vi "Secondary Moniter.vi"() -> ()   [LabVIEW 2018]
uses:
  <vilib>/Rock Robotics/Network Tables/NT Read Number.vi
  <vilib>/Rock Robotics/Network Tables/NT Read Boolean.vi
  <vilib>/Rock Robotics/Network Tables/NT Read Boolean Array.vi
panel:
  out "Boolean 10":bool
  out "Boolean 9":bool
  out "Boolean 8":bool
  out "Boolean 7":bool
  out "Boolean 6":bool
  out "Boolean 5":bool
  out "Boolean 4":bool
  out "Boolean 3":bool
  out "Boolean 2":bool
  out "Boolean":bool
  out "XY Graph":cluster{"Y":dbl[], "Y":dbl[]}[](graph)
  out "Low Gear":bool
  out "High Gear":bool
  out "Climber":bool
  out "Robot Centric":bool
  out "Field Centric":bool
  out "Tracks":bool caption="Brakes"
  out "Match Time":string
  out "Camera Image 2":T1(plugin-control)
  out "PSI":dbl(slide) scale=0.0..160.0
  out "Gyro":cluster{dbl, dbl}(knob) scale=0.0..360.0 scale format="%#.3g"
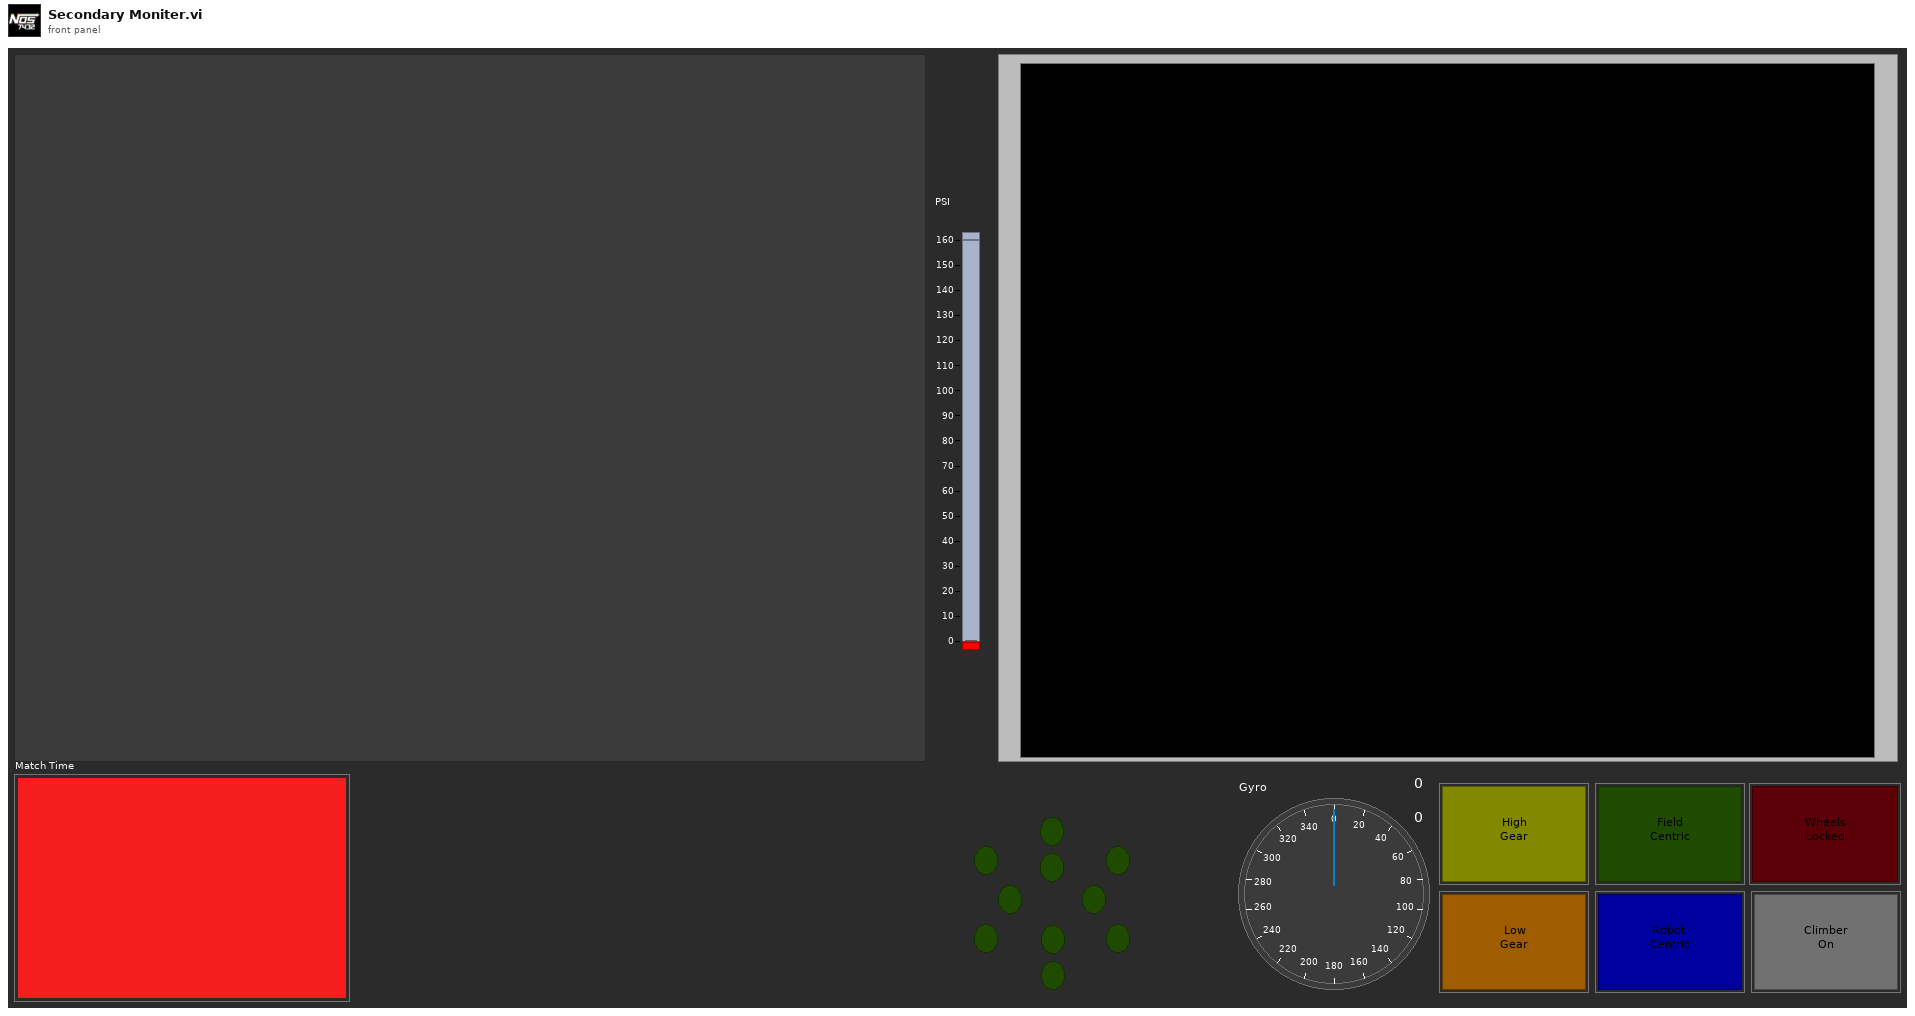
[diagram p1: front panel]
types:
  T1 = typedef "IMAQ Image.ctl" = refnum<image>
  T2 = typedef "LVDateTimeRec.ctl" = cluster{"fractional second":dbl, "second":i32, "minute":i32, "hour":i32, "day of month":i32, "month":i32, "year":i32, "day of week":i32, "day of year":i32, "DST":i32}
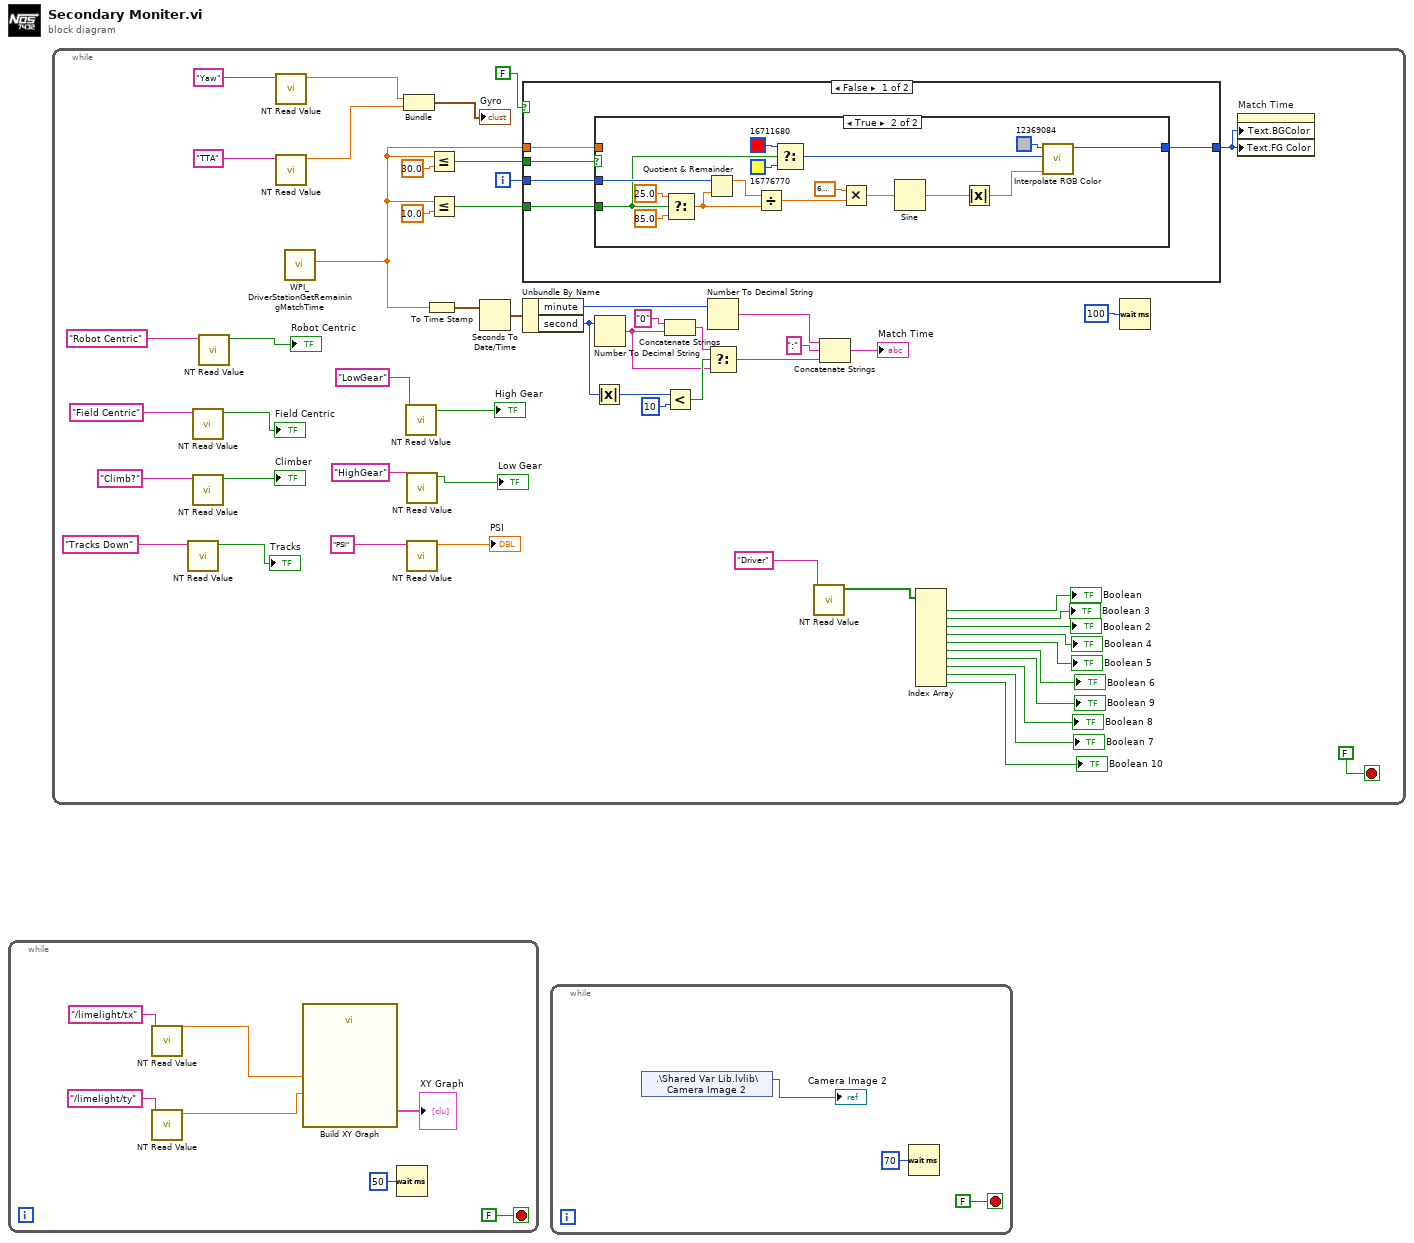
[diagram p0: block diagram]
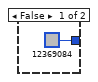
[diagram p2: hidden frame]
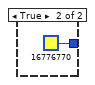
[diagram p3: hidden frame]
diagram:
  n1 = while {
    stop <- FALSE stop-if-true
    n2 = call-poly <vilib>:"NT Read Value.vi"("Name"="/limelight/tx") -> ("Numeric"=w4:dbl)  [unwired: 9 in, 1 out]
    n3 = call-poly <vilib>:"NT Read Value.vi"("Name"="/limelight/ty") -> ("Numeric"=w3:dbl)  [unwired: 9 in, 1 out]
    n4 = call "Build XY Graph"("Y Input"=w3, "X Input"=w4) -> ("XY Graph"=→"XY Graph":cluster{"X":dbl[], "Y":dbl[]}[])  [unwired: 8 in, 1 out]
    n5 = Wait (ms)(milliseconds to wait=u32 50) -> ()  [unwired: 1 out]
  }
  n6 = while {
    i -> [w40]
    stop <- FALSE stop-if-true
    n7 = call-poly <vilib>:"NT Read Value.vi"("Name"="Tracks Down") -> ("Boolean"=→"Tracks":bool)  [unwired: 9 in, 1 out]
    n8 = call-poly <vilib>:"NT Read Value.vi"("Name"="Field Centric") -> ("Boolean"=→"Field Centric":bool)  [unwired: 9 in, 1 out]
    n9 = call-poly <vilib>:"NT Read Value.vi"("Name"="Climb?") -> ("Boolean"=→"Climber":bool)  [unwired: 9 in, 1 out]
    n10 = call-poly <vilib>:"NT Read Value.vi"("Name"="Robot Centric") -> ("Boolean"=→"Robot Centric":bool)  [unwired: 9 in, 1 out]
    n11 = call-poly <vilib>:"NT Read Value.vi"("Name"="Yaw") -> ("Numeric"=w21:dbl)  [unwired: 9 in, 1 out]
    n12 = call-poly <vilib>:"NT Read Value.vi"("Name"="TTA") -> ("Numeric"=w22:dbl)  [unwired: 9 in, 1 out]
    n13 = call <vilib>:"WPI_DriverStationGetRemainingMatchTime.vi"() -> ("Match Time(s)"=w32:sgl)  [unwired: 10 in, 1 out]
    n14 = Bundle("Numeric"=w21, "Numeric"=w22) -> (→"Gyro":cluster{"Numeric":dbl, "Numeric":dbl})  [unwired: 1 in]
    n15 = call-poly <vilib>:"NT Read Value.vi"("Name"="LowGear") -> ("Boolean"=→"High Gear":bool)  [unwired: 9 in, 1 out]
    n16 = call-poly <vilib>:"NT Read Value.vi"("Name"="HighGear") -> ("Boolean"=→"Low Gear":bool)  [unwired: 9 in, 1 out]
    n17 = call-poly <vilib>:"NT Read Value.vi"("Name"="PSI") -> ("Numeric"=→"PSI":dbl)  [unwired: 9 in, 1 out]
    n18 = To Time Stamp(1:w32) -> (0:w41:timestamp)
    n19 = Less Or Equal?(x=w32, y=30.0) -> (x <= y?=w36:bool)
    n20 = Less Or Equal?(x=w32, y=10.0) -> (x <= y?=w37:bool)
    n21 = Seconds To Date/Time(time stamp (now)=w41) -> (date time rec=w34:T2)  [unwired: 1 in]
    n22 = case shown="False" FALSE {
      tunnel: w36 -> [w67 _]
      tunnel: w37 -> [w66 _]
      tunnel: [w65 u32 16776770 ("Color")] -> w35
      tunnel: w32 -> [w64 _]
      tunnel: w40 -> [w63 _]
      frame False {
        n23 = case shown="True" w67 {
          tunnel: w66 -> [_ w72]
          tunnel: [u32 12369084 ("Color") w73] -> w65
          tunnel: w64 -> [_ _]
          tunnel: w63 -> [_ w76]
          frame False {
          }
          frame True {
            n24 = Select(t=25.0, s=w72, f=85.0) -> (s? t:f=w69:dbl)
            n25 = Quotient & Remainder(x=w76, y=w69) -> (x-y*floor(x/y)=w79:dbl)  [unwired: 1 out]
            n26 = Divide(x=w79, y=w69) -> (x/y=w78:dbl)
            n27 = Select(t=u32 16711680 ("Color"), s=w72, f=u32 16776770 ("Color")) -> (s? t:f=w75:u32)
            n28 = Multiply(x=6.283185307179586, y=w78) -> (x*y=w81:dbl)
            n29 = Sine(x=w81) -> (sin(x)=w80:dbl)
            n30 = Absolute Value(x=w80) -> (abs(x)=w77:dbl)
            n31 = call "Interpolate RGB Color.vi"("Proportion"=w77, "Target Color"=w75, "Base Color"=u32 12369084 ("Color")) -> ("Result Color"=w73:u32)  [unwired: 8 in]
          }
        }
      }
      frame True {
      }
    }
    n32 = Unbundle By Name(w34) -> ("minute"=w42:i32, "second"=w43:i32)
    n33 = Absolute Value(x=w43) -> (abs(x)=w51:i32)
    n34 = Number To Decimal String(number=w43) -> (decimal integer string=w46:string)  [unwired: 1 in]
    n35 = Concatenate Strings("0" ("string"), w46) -> (w48:string)
    n36 = Less?(x=w51, y=10) -> (x < y?=w47:bool)
    n37 = Number To Decimal String(number=w42) -> (decimal integer string=w52:string)  [unwired: 1 in]
    n38 = Select(t=w48, s=w47, f=w46) -> (s? t:f=w45:string)
    n39 = call-poly <vilib>:"NT Read Value.vi"("Name"="Driver") -> ("Boolean Array"=w18:bool[])  [unwired: 9 in, 1 out]
    n40 = Concatenate Strings(w52, ":" ("string"), w45) -> (→"Match Time":string)
    n41 = Index Array(array=w18) -> (element #1=→"Boolean":bool, element #2=→"Boolean 3":bool, element #3=→"Boolean 2":bool, element #4=→"Boolean 4":bool, element #5=→"Boolean 5":bool, element #6=→"Boolean 6":bool, element #7=→"Boolean 9":bool, element #8=→"Boolean 8":bool, element #9=→"Boolean 7":bool, element #10=→"Boolean 10":bool)  [unwired: 10 in]
    n42 = Wait (ms)(milliseconds to wait=u32 100) -> ()  [unwired: 1 out]
    n43 = property on="Match Time" class="Str"("Text.BGColor"=w35, "Text.FG Color"=w35) -> ()  [unwired: 2 in, 2 out]
  }
  n44 = while {
    stop <- FALSE stop-if-true
    n45 = shared-variable ".\\Shared Var Lib.lvlib\\Camera Image 2"() -> (→"Camera Image 2":refnum<image>)  [unwired: 1 in, 1 out]
    n46 = Wait (ms)(milliseconds to wait=u32 70) -> ()  [unwired: 1 out]
  }
